vi "Acquire Continuously.vi"(8 "error in (no error)":errorcluster, 11 "Measurement in":refnum<class "Measurement.lvclass">) -> (0 "error out":errorcluster, 3 "Measurement out":refnum<class "Measurement.lvclass">)   [LabVIEW 2016, in "Measurement Actor.lvlib" / "Measurement.lvclass"]
uses:
  Measurement.lvclass
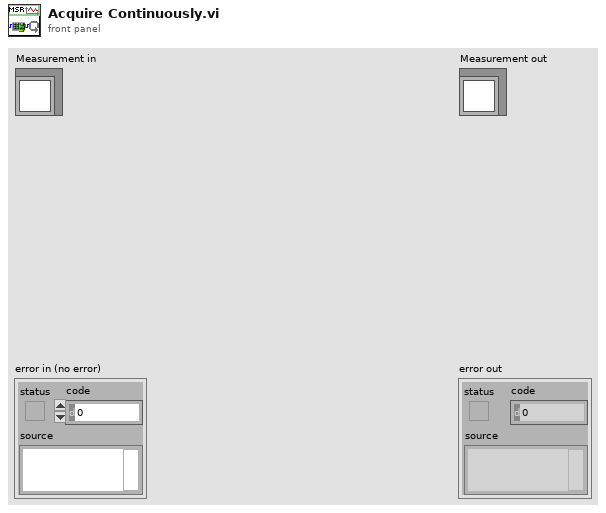
[diagram p1: front panel]
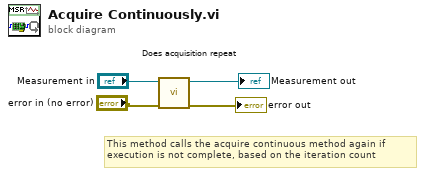
[diagram p0: block diagram]
diagram:
  # "This method calls the acquire continuous method again if \nexecution is not complete, based on the iteration count"
  n1 = call "Does acquisition repeat.vi"("error in (no error)"="error in (no error)", "Measurement in"="Measurement in") -> ("error out"=→"error out":errorcluster, "Measurement out"=→"Measurement out":refnum<class "Measurement.lvclass">)  [unwired: 8 in]
